vi "Read Analyze Objects.vi"(8 "error in (no error)":errorcluster, 11 "Analyze Actor in":refnum<class "Analyze Actor.lvclass">) -> (0 "error out":errorcluster, 2 "Analyze Objects":refnum<class "Analyze BaseClass.lvclass">[](array[class]), 3 "Analyze Actor out":refnum<class "Analyze Actor.lvclass">)   [LabVIEW 2020]
uses:
  Analyze Actor.lvclass
  Analyze Classes/Analyze BaseClass/Analyze BaseClass/Analyze BaseClass.lvclass
  Analyze Actor.lvclass/Analyze Actor.ctl
  C:/Program Files (x86)/National Instruments/LabVIEW 2020/vi.lib/ActorFramework/Actor/Actor.lvclass
  C:/Users/AlexK/work/LabVIEW Programme/POLARIS-AS-3-Cams/Submodules/HIJ Vision/Analyze/Analyze Actor/Analyze Actor/Analyze Actor.lvclass
  C:/Users/AlexK/work/LabVIEW Programme/POLARIS-AS-3-Cams/Submodules/HIJ Vision/Analyze/Analyze Classes/Analyze BaseClass/Analyze BaseClass/Analyze BaseClass.lvclass
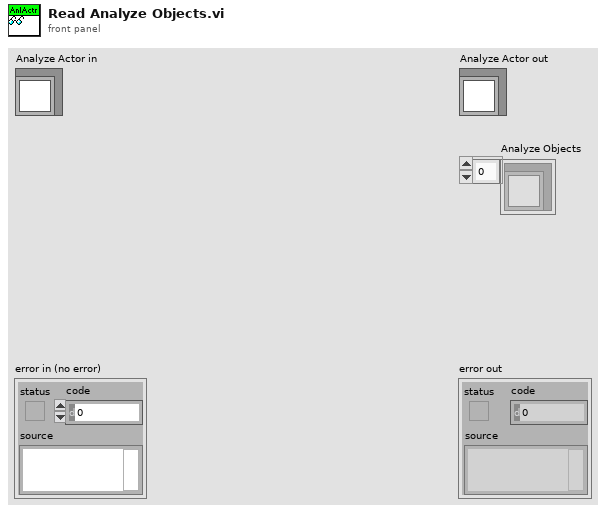
[diagram p1: front panel]
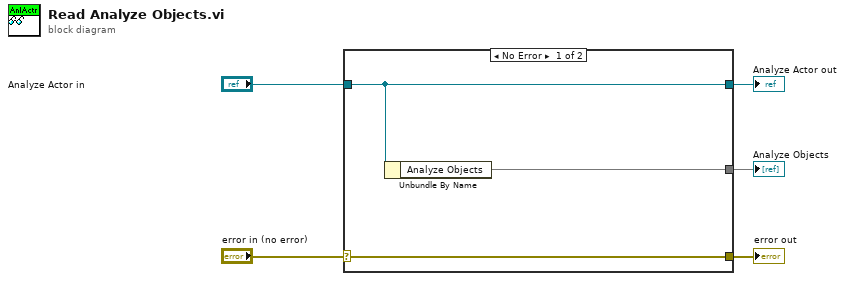
[diagram p0: block diagram]
diagram:
  n1 = case shown="No Error" "error in (no error)" {
    selector: "error in (no error)" -> [w8 w9]
    tunnel: [w8 w9] -> w4
    tunnel: [w7 w10] -> w2
    tunnel: "Analyze Actor in" -> [w7 w10]
    tunnel: [w6 _] -> w1
    frame No Error {
      n2 = Unbundle By Name(w7) -> ("Analyze Objects"=w6)
    }
    frame Error {
    }
  }
  "error out" <- w4
  "Analyze Actor out" <- w2
  "Analyze Objects" <- w1
